vi "PWM RT1.vi"(10 "占空比":ext, 11 "频率":u16) -> (3 "PWM FT":u32)   [LabVIEW 2017]
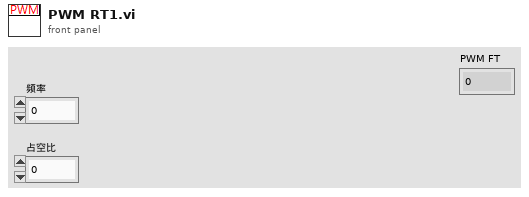
[diagram p1: front panel]
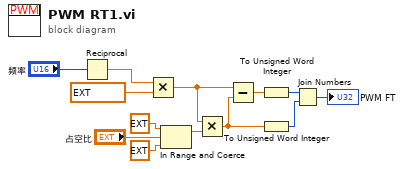
[diagram p0: block diagram]
diagram:
  n1 = Reciprocal ("倒数")(x="频率") -> (1/x=w11:ext)
  n2 = Multiply(x=w11, y=ext 1000000.0) -> (x*y=w13:ext)
  n3 = In Range and Coerce(upper limit=ext 1.0 ("上限"), x="占空比", lower limit=ext 0.0 ("下限")) -> (coerced(x)=w1:ext)  [unwired: 1 out]
  n4 = Multiply(x=w13, y=w1) -> (x*y=w5:ext)
  n5 = Subtract(x=w13, y=w5) -> (x-y=w6:ext)
  n6 = To Unsigned Word Integer(number=w6) -> (unsigned 16bit integer=w4:u16)
  n7 = To Unsigned Word Integer(number=w5) -> (unsigned 16bit integer=w3:u16)
  n8 = Join Numbers(hi=w4, lo=w3) -> ((hi.lo)=→"PWM FT":u32)
